vi "Convert QD Object String to 2D Array.vi"(11 "objects string":string) -> (2 "already sorted":bool, 3 "objects 2D array":string[][](array[string]))   [LabVIEW 2024]
uses:
  QD Suggestion.ctl
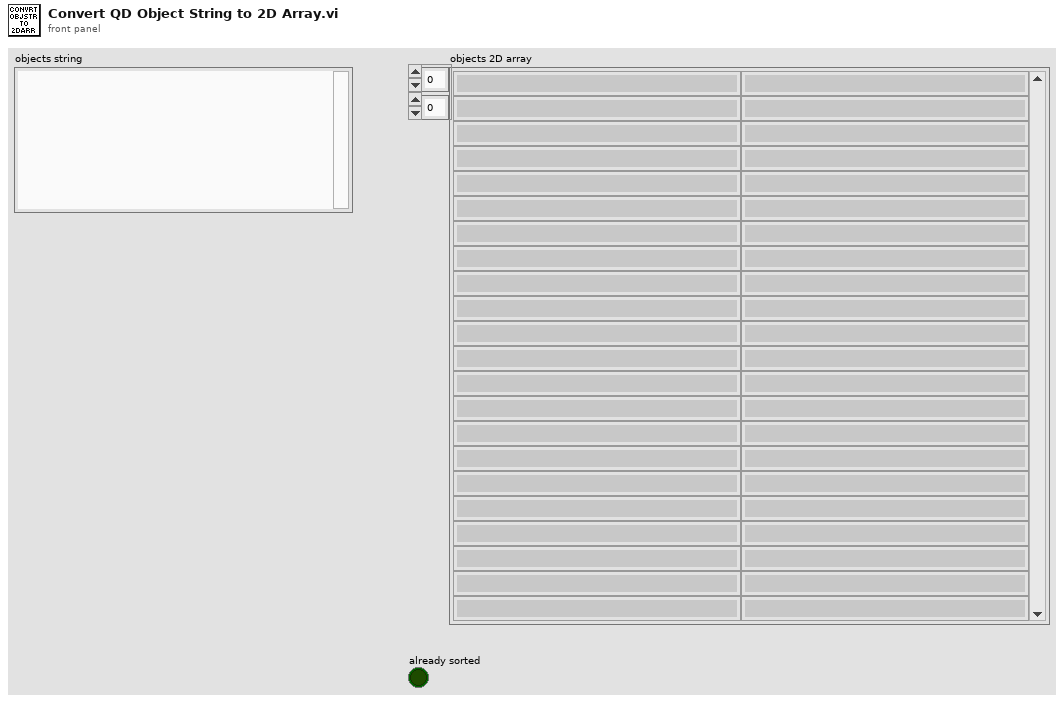
[diagram p1: front panel]
types:
  T1 = typedef "QD Suggestion.ctl" = cluster{"Data":string, "qd":string[], "Type":string}
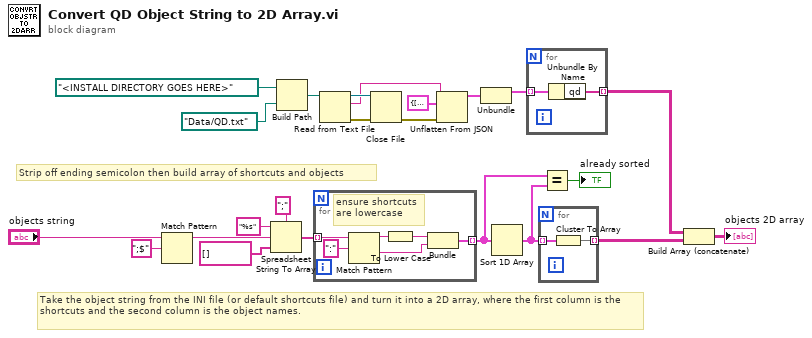
[diagram p0: block diagram]
diagram:
  # "Take the object string from the INI file (or default shortcuts file) and turn it into a 2D array, where the first column is the shortcuts and the second column is the object names."
  # "Strip off ending semicolon then build array of shortcuts and objects"
  n1 = Match Pattern(string="objects string", regular expression=";$") -> (before substring=w23:string)  [unwired: 1 in, 3 out]
  n2 = Spreadsheet String To Array(delimiter (Tab)=";", format string="%s", spreadsheet string=w23, array type (2D Dbl)=string[] []) -> (array=w19:string[])
  n3 = Build Path(base path=path "<INSTALL DIRECTORY GOES HERE>", name or relative path=path "Data/QD.txt" ("file (use dialog)")) -> (appended path=w3:path)
  n4 = for {
    tunnel: w19 -> [w29] mode=indexing
    tunnel: [w24] -> w16 mode=indexing
    # "ensure shortcuts\nare lowercase"
    n5 = Match Pattern(string=w29, regular expression=":") -> (before substring=w27:string, after substring=w25:string)  [unwired: 1 in, 2 out]
    n6 = To Lower Case(string=w27) -> (all lower case string=w26:string)
    n7 = Bundle(w26, w25) -> (w24:cluster{string, string})  [unwired: 1 in]
  }
  n8 = Read from Text File(file (use dialog)=w3) -> (refnum out=w13:refnum<file>, text=w11:string, error out=w12:errorcluster)  [unwired: 3 in, 1 out]
  n9 = Close File(refnum=w13, error in=w12) -> (error out=w8:errorcluster)  [unwired: 1 out]
  n10 = Unflatten From JSON(JSON string=w11, type and defaults=cluster{T1[], cluster{"Left":i32, "Top":i32}} {[], {"Left"=0, "Top"=0}} ("cluster"), error in (no error)=w8) -> (value=w5:cluster{T1[], cluster{"Left":i32, "Top":i32}})  [unwired: 4 in, 1 out]
  n11 = Unbundle(w5) -> (w4:T1[])  [unwired: 1 out]
  n12 = Sort 1D Array(array=w16) -> (sorted array=w15:cluster{string, string}[])
  n13 = for {
    tunnel: w4 -> [w31] mode=indexing
    tunnel: [w30] -> w7 mode=indexing
    n14 = Unbundle By Name(w31) -> ("qd"=w30:string[])
  }
  n15 = for {
    tunnel: w15 -> [w33] mode=indexing
    tunnel: [w32] -> w10 mode=indexing
    n16 = Cluster To Array(cluster=w33) -> (array=w32:string[])
  }
  n17 = Equal?(x=w16, y=w15) -> (x = y?=→"already sorted":bool)
  n18 = Build Array (concatenate)(w7, w10) -> (→"objects 2D array":string[][])
